vi "AVI file path manager core.vi"(8 "error in (no error)":errorcluster, 10 "Value in":path, 11 "Path in":refnum<vi>) -> (0 "error out":errorcluster, 2 "File path OK":bool, 3 "File path":path)   [LabVIEW 2020]
uses:
  Globals/gl_Time series viewer globals.vi
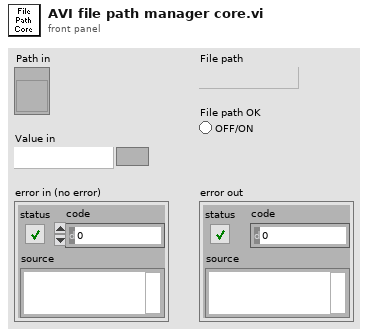
[diagram p1: front panel]
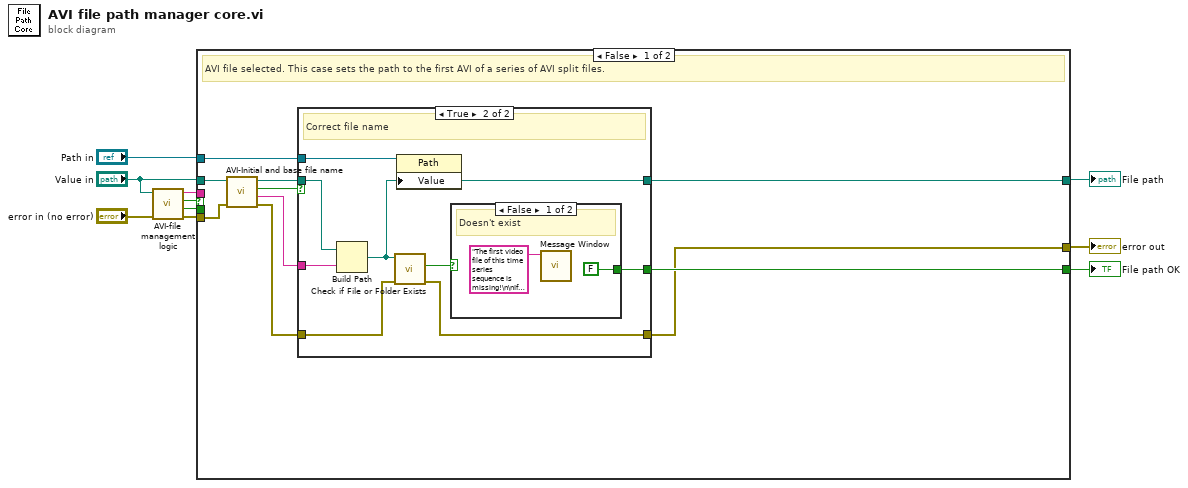
[diagram p0: block diagram]
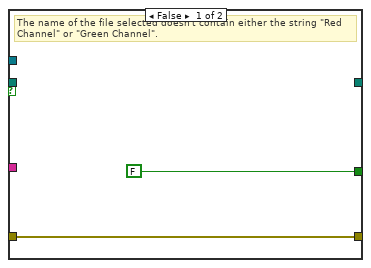
[diagram p2: hidden frame]
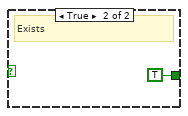
[diagram p3: hidden frame]
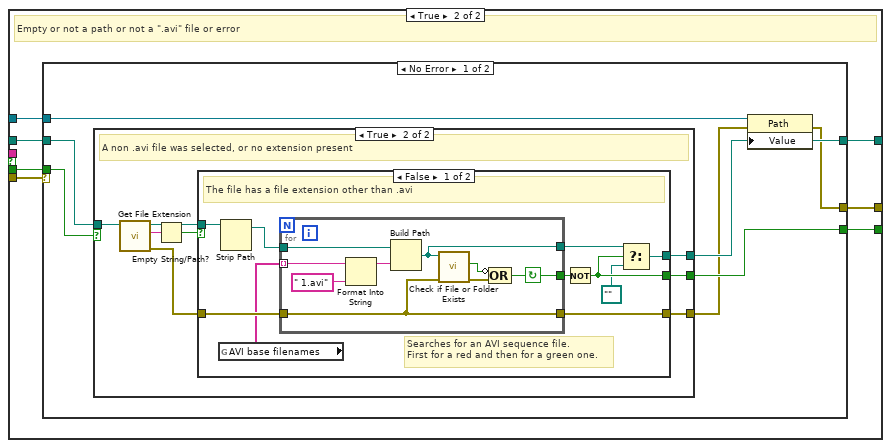
[diagram p4: hidden frame]
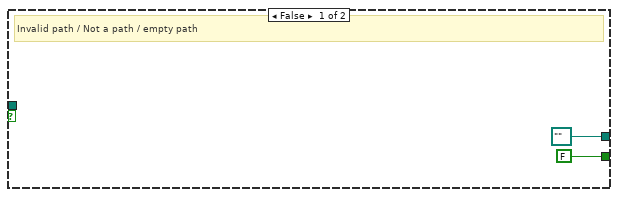
[diagram p5: hidden frame]
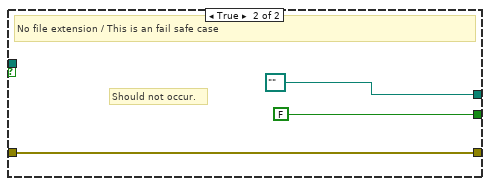
[diagram p6: hidden frame]
diagram:
  n1 = call "AVI-file management logic.vi"("error in (no error)"="error in (no error)", "First AVI2 video's Path"="Value in") -> ("error out"=w8:errorcluster, "A non .avi file was selected, or no extension present"=w6:bool, "Empty or not a path or not a \".avi\" file or error"=w4:bool, "filename without extension"=w5:string)  [unwired: 6 in]
  n2 = case shown="False" w4 {
    tunnel: [w18 w40] -> w1
    tunnel: "Value in" -> [w16 w37]
    tunnel: [w19 w38] -> w3
    tunnel: "Path in" -> [w17 w39]
    tunnel: w5 -> [_ _]
    tunnel: w6 -> [_ w36]
    tunnel: w8 -> [w14 w34]
    tunnel: [w12 w35] -> w9
    frame False {
      # "AVI file selected. This case sets the path to the first AVI of a series of AVI split files."
      n3 = call "AVI-Initial and base file name.vi"("error in (no error)"=w14, "AVI file path & name"=w16) -> ("error out"=w13:errorcluster, "Initial file name (increment = 1)"=w11:string, "Base name is valid"=w20:bool, "AVI file path"=w15:path)  [unwired: 5 in, 1 out]
      n4 = case shown="True" w20 {
        tunnel: [FALSE ("File path OK") w26] -> w18
        tunnel: w15 -> [_ w30]
        tunnel: [_ w28] -> w19
        tunnel: w17 -> [_ w29]
        tunnel: w13 -> [w21 w25]
        tunnel: [w21 w24] -> w12
        tunnel: w11 -> [_ w23]
        frame False {
          # "The name of the file selected doesn't contain either the string \"Red Channel\" or \"Green Channel\"."
        }
        frame True {
          # "Correct file name"
          n5 = Build Path(base path=w30, name or relative path=w23) -> (appended path=w28:path)
          n6 = call <vilib>:"Check if File or Folder Exists.vi"("error in (no error)"=w25, "path"=w28) -> ("error out"=w24:errorcluster, "file or folder exists?"=w27:bool)  [unwired: 7 in, 1 out]
          n7 = property class="Path"(reference=w29, "Value"=w28) -> ()  [unwired: 1 in, 2 out]
          n8 = case shown="False" w27 {
            tunnel: [FALSE TRUE] -> w26
            frame False {
              # "Doesn't exist"
              n9 = call "Message Window.vi"("Message string"="The first video file of this time series sequence is missing!\n\nIf you want to play the file you selected rename it to \"Red Channel 1\" or \"Green Channel 1\" and try re-loading it.") -> ()  [unwired: 10 in, 1 out]
            }
            frame True {
              # "Exists"
            }
          }
        }
      }
    }
    frame True {
      # "Empty or not a path or not a \".avi\" file or error"
      n10 = case shown="No Error" w34 {
        selector: w34 -> [_ w80]
        tunnel: [w47 _] -> w40
        tunnel: w39 -> [w46 _]
        tunnel: [w45 w81] -> w38
        tunnel: w37 -> [w44 w81]
        tunnel: w36 -> [w43 _]
        tunnel: [w41 w80] -> w35
        frame No Error {
          n11 = case shown="True" w43 {
            tunnel: [FALSE ("File path OK 2") w54] -> w47
            tunnel: [path "" ("Value") w53] -> w45
            tunnel: w44 -> [_ w57]
            tunnel: [_ w50] -> w42
            frame False {
              # "Invalid path / Not a path / empty path"
            }
            frame True {
              # "A non .avi file was selected, or no extension present"
              n12 = call <vilib>:"Get File Extension.vi"("file"=w57) -> ("error out"=w51:errorcluster, "lowercase file extension"=w56:string, "dup file"=w52:path)  [unwired: 6 in, 2 out]
              n13 = Empty String/Path?(string/path=w56) -> (empty?=w55:bool)
              n14 = case shown="False" w55 {
                tunnel: [w64 FALSE ("File path OK 2")] -> w54
                tunnel: [w62 path "" ("Value")] -> w53
                tunnel: w52 -> [w67 _]
                tunnel: w51 -> [w60 w77]
                tunnel: [w59 w77] -> w50
                frame False {
                  # "Searches for an AVI sequence file.\nFirst for a red and then for a green one."
                  # "The file has a file extension other than .avi"
                  n15 = global read "gl_Time series viewer globals.vi" "AVI base filenames"() -> (w58:string[])
                  n16 = Strip Path(path=w67) -> (stripped path=w66:path)  [unwired: 1 out]
                  n17 = for {
                    tunnel: w58 -> [w75] mode=indexing
                    tunnel: w66 -> [w74]
                    tunnel: [w70] -> w65
                    tunnel: [w69] -> w63
                    tunnel: w60 -> [w68]
                    tunnel: [w68] -> w59
                    stop <- w70 continue-if-true
                    n18 = Format Into String(initial string=w75, " 1.avi" ("format string")) -> (resulting string=w73:string)  [unwired: 2 in, 1 out]
                    n19 = Build Path(base path=w74, name or relative path=w73) -> (appended path=w69:path)
                    n20 = call <vilib>:"Check if File or Folder Exists.vi"("error in (no error)"=w68, "path"=w69) -> ("error out"=w72:errorcluster, "file or folder exists?"=w71:bool)  [unwired: 7 in, 1 out]
                    n21 = Compound Arithmetic op=OR(invert w71, w72) -> (w70:bool)
                  }
                  n22 = Not(x=w65) -> (.not. x?=w64:bool)
                  n23 = Select(t=w63, s=w64, f=path "" ("Value")) -> (s? t:f=w62:path)
                }
                frame True {
                  # "Should not occur."
                  # "No file extension / This is an fail safe case"
                }
              }
            }
          }
          n24 = property class="Path"(reference=w46, error in=w42, "Value"=w45) -> (error out=w41:errorcluster)  [unwired: 1 out]
        }
        frame Error {
        }
      }
    }
  }
  "error out" <- w9
  "File path" <- w3
  "File path OK" <- w1
